vi "Control Channels.vi"(8 "error in (no error)":errorcluster, 10 "Array":dbl[](array[numeric]), 11 "IVI Refnum in":refnum<k15>) -> (0 "error out":errorcluster, 3 "IVI Refnum out":refnum<k15>)   [LabVIEW 2020, in "PXI-2514 Engine.lvlib"]
uses:
  PXI-2514 Engine.lvlib
  <instrlib>/niSwitch/niSwitch.llb/niSwitch Relay Action.ctl
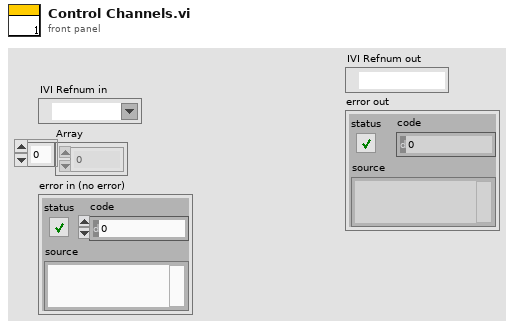
[diagram p1: front panel]
types:
  T1 = enum16{"Default", "DUT Pass Through", "DUT Open", "DUT Pass Through and FB A", "DUT Pass Through and FB B", "DUT FB A", "DUT FB B"}
  T2 = typedef "niSwitch Relay Action.ctl" = i32
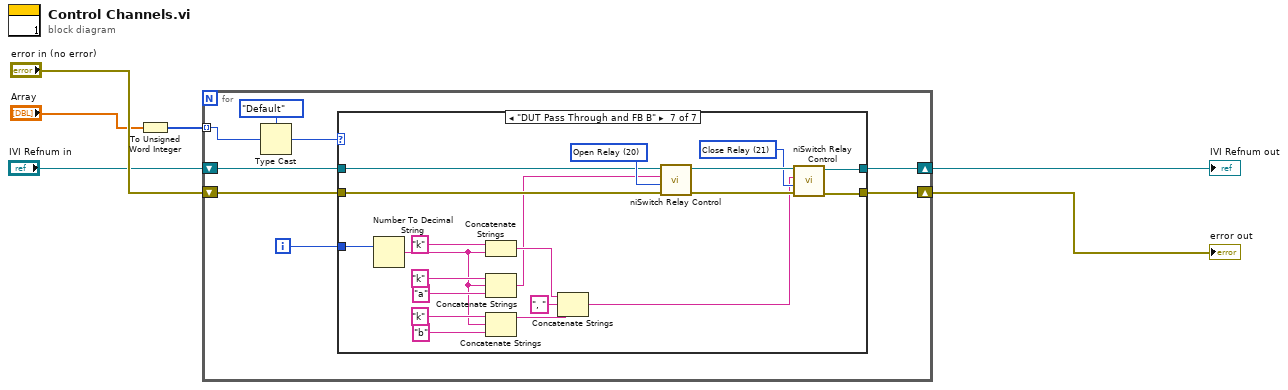
[diagram p0: block diagram]
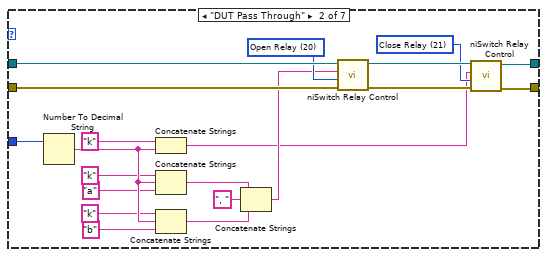
[diagram p3: hidden frame]
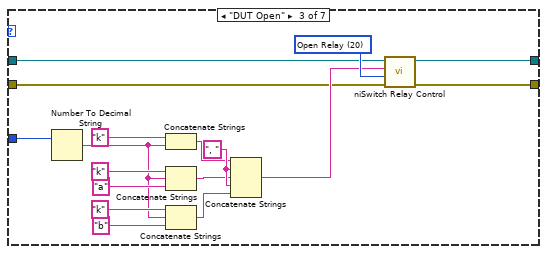
[diagram p4: hidden frame]
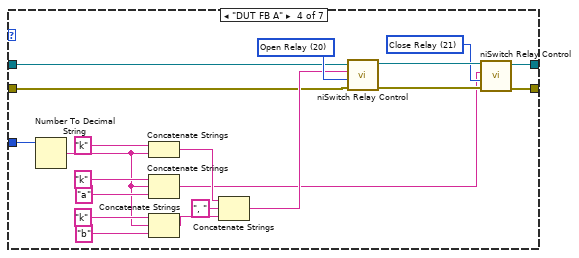
[diagram p5: hidden frame]
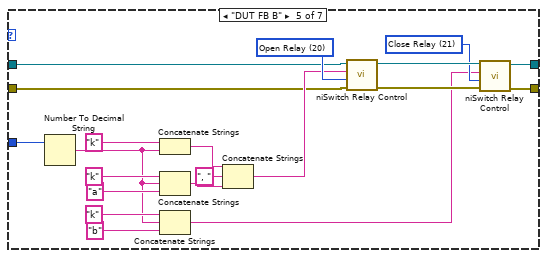
[diagram p6: hidden frame]
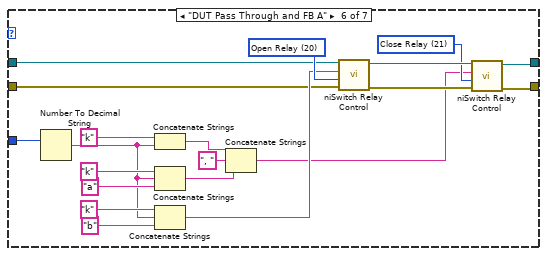
[diagram p7: hidden frame]
diagram:
  n1 = To Unsigned Word Integer(number="Array") -> (unsigned 16bit integer=w3:u16[])
  n2 = for {
    tunnel: w3 -> [w11] mode=indexing
    shift-right: [w9] -> w2
    shift-left: "IVI Refnum in" -> [w13]
    shift-right: [w8] -> w1
    shift-left: "error in (no error)" -> [w14]
    i -> [w7]
    n3 = Type Cast(type=T1."Default", x=w11) -> (*(type *) &x=w10:T1)
    n4 = case shown="\"DUT Pass Through and FB B\"" w10 {
      tunnel: w14 -> [w15 w36 w38 w54 w77 w94 w116]
      tunnel: w13 -> [w16 w35 w40 w55 w76 w95 w117]
      tunnel: [w16 w24 w41 w56 w74 w96 w119] -> w9
      tunnel: [w15 w25 w37 w57 w75 w97 w118] -> w8
      tunnel: w7 -> [_ w17 w43 w64 w84 w104 w124]
      frame "Default", Default {
      }
      frame "DUT Pass Through" {
        w20 = T2 21 items=["Open Relay"=20, "Close Relay"=21] ("relay action (Close Relay)")
        w21 = T2 20 items=["Open Relay"=20, "Close Relay"=21] ("relay action (Close Relay)")
        n5 = Number To Decimal String(number=w17) -> (decimal integer string=w33:string)  [unwired: 1 out]
        n6 = Concatenate Strings("k", w33) -> (w18:string)
        n7 = Concatenate Strings("k", w33, "a") -> (w27:string)
        n8 = Concatenate Strings("k", w33, "b") -> (w26:string)
        n9 = Concatenate Strings(w27, ", " ("string"), w26) -> (w19:string)
        n10 = call <instrlib>:"niSwitch Relay Control.vi"("error in (no error)"=w36, "relay action (Close Relay)"=w21, "relay names"=w19, "instrument handle"=w35) -> ("error out"=w22:errorcluster, "instrument handle out"=w23:refnum<k15>)  [unwired: 6 in]
        n11 = call <instrlib>:"niSwitch Relay Control.vi"("error in (no error)"=w22, "relay action (Close Relay)"=w20, "relay names"=w18, "instrument handle"=w23) -> ("error out"=w25:errorcluster, "instrument handle out"=w24:refnum<k15>)  [unwired: 6 in]
      }
      frame "DUT Open" {
        w42 = T2 20 items=["Open Relay"=20, "Close Relay"=21] ("relay action (Close Relay)")
        w53 = ", " ("string")
        n12 = Number To Decimal String(number=w43) -> (decimal integer string=w44:string)  [unwired: 1 out]
        n13 = Concatenate Strings("k", w44) -> (w47:string)
        n14 = Concatenate Strings("k", w44, "a") -> (w46:string)
        n15 = Concatenate Strings("k", w44, "b") -> (w45:string)
        n16 = Concatenate Strings(w47, w53, w46, w53, w45) -> (w39:string)
        n17 = call <instrlib>:"niSwitch Relay Control.vi"("error in (no error)"=w38, "relay action (Close Relay)"=w42, "relay names"=w39, "instrument handle"=w40) -> ("error out"=w37:errorcluster, "instrument handle out"=w41:refnum<k15>)  [unwired: 6 in]
      }
      frame "DUT FB A" {
        w60 = T2 21 items=["Open Relay"=20, "Close Relay"=21] ("relay action (Close Relay)")
        w61 = T2 20 items=["Open Relay"=20, "Close Relay"=21] ("relay action (Close Relay)")
        n18 = Number To Decimal String(number=w64) -> (decimal integer string=w67:string)  [unwired: 1 out]
        n19 = Concatenate Strings("k", w67) -> (w66:string)
        n20 = Concatenate Strings("k", w67, "a") -> (w58:string)
        n21 = Concatenate Strings("k", w67, "b") -> (w65:string)
        n22 = Concatenate Strings(w66, ", " ("string"), w65) -> (w59:string)
        n23 = call <instrlib>:"niSwitch Relay Control.vi"("error in (no error)"=w54, "relay action (Close Relay)"=w61, "relay names"=w59, "instrument handle"=w55) -> ("error out"=w62:errorcluster, "instrument handle out"=w63:refnum<k15>)  [unwired: 6 in]
        n24 = call <instrlib>:"niSwitch Relay Control.vi"("error in (no error)"=w62, "relay action (Close Relay)"=w60, "relay names"=w58, "instrument handle"=w63) -> ("error out"=w57:errorcluster, "instrument handle out"=w56:refnum<k15>)  [unwired: 6 in]
      }
      frame "DUT FB B" {
        w80 = T2 21 items=["Open Relay"=20, "Close Relay"=21] ("relay action (Close Relay)")
        w81 = T2 20 items=["Open Relay"=20, "Close Relay"=21] ("relay action (Close Relay)")
        n25 = Number To Decimal String(number=w84) -> (decimal integer string=w87:string)  [unwired: 1 out]
        n26 = Concatenate Strings("k", w87) -> (w86:string)
        n27 = Concatenate Strings("k", w87, "a") -> (w85:string)
        n28 = Concatenate Strings("k", w87, "b") -> (w78:string)
        n29 = Concatenate Strings(w86, ", " ("string"), w85) -> (w79:string)
        n30 = call <instrlib>:"niSwitch Relay Control.vi"("error in (no error)"=w77, "relay action (Close Relay)"=w81, "relay names"=w79, "instrument handle"=w76) -> ("error out"=w82:errorcluster, "instrument handle out"=w83:refnum<k15>)  [unwired: 6 in]
        n31 = call <instrlib>:"niSwitch Relay Control.vi"("error in (no error)"=w82, "relay action (Close Relay)"=w80, "relay names"=w78, "instrument handle"=w83) -> ("error out"=w75:errorcluster, "instrument handle out"=w74:refnum<k15>)  [unwired: 6 in]
      }
      frame "DUT Pass Through and FB A" {
        w100 = T2 21 items=["Open Relay"=20, "Close Relay"=21] ("relay action (Close Relay)")
        w101 = T2 20 items=["Open Relay"=20, "Close Relay"=21] ("relay action (Close Relay)")
        n32 = Number To Decimal String(number=w104) -> (decimal integer string=w107:string)  [unwired: 1 out]
        n33 = Concatenate Strings("k", w107) -> (w106:string)
        n34 = Concatenate Strings("k", w107, "a") -> (w105:string)
        n35 = Concatenate Strings("k", w107, "b") -> (w99:string)
        n36 = Concatenate Strings(w106, ", " ("string"), w105) -> (w98:string)
        n37 = call <instrlib>:"niSwitch Relay Control.vi"("error in (no error)"=w94, "relay action (Close Relay)"=w101, "relay names"=w99, "instrument handle"=w95) -> ("error out"=w102:errorcluster, "instrument handle out"=w103:refnum<k15>)  [unwired: 6 in]
        n38 = call <instrlib>:"niSwitch Relay Control.vi"("error in (no error)"=w102, "relay action (Close Relay)"=w100, "relay names"=w98, "instrument handle"=w103) -> ("error out"=w97:errorcluster, "instrument handle out"=w96:refnum<k15>)  [unwired: 6 in]
      }
      frame "DUT Pass Through and FB B" {
        w120 = T2 21 items=["Open Relay"=20, "Close Relay"=21] ("relay action (Close Relay)")
        w121 = T2 20 items=["Open Relay"=20, "Close Relay"=21] ("relay action (Close Relay)")
        n39 = Number To Decimal String(number=w124) -> (decimal integer string=w127:string)  [unwired: 1 out]
        n40 = Concatenate Strings("k", w127) -> (w126:string)
        n41 = Concatenate Strings("k", w127, "a") -> (w114:string)
        n42 = Concatenate Strings("k", w127, "b") -> (w125:string)
        n43 = Concatenate Strings(w126, ", " ("string"), w125) -> (w115:string)
        n44 = call <instrlib>:"niSwitch Relay Control.vi"("error in (no error)"=w116, "relay action (Close Relay)"=w121, "relay names"=w114, "instrument handle"=w117) -> ("error out"=w122:errorcluster, "instrument handle out"=w123:refnum<k15>)  [unwired: 6 in]
        n45 = call <instrlib>:"niSwitch Relay Control.vi"("error in (no error)"=w122, "relay action (Close Relay)"=w120, "relay names"=w115, "instrument handle"=w123) -> ("error out"=w118:errorcluster, "instrument handle out"=w119:refnum<k15>)  [unwired: 6 in]
      }
    }
  }
  "IVI Refnum out" <- w2
  "error out" <- w1
